vi "build data packet.vi"(0 "Priority (Act immediately)":u8(ring) items=["Act immediately", "Act immediately but disregard errors", "Do not process"], 5 "Timestamp (now)":timestamp, 7 "Metadata":u8[](array[numeric]), 9 "DATA":u8[](array[numeric]), 11 "Footer":u8[](array[numeric])) -> (4 "Byte array":u8[](array[numeric]))   [LabVIEW 2020, in "Template.lvlib" / "Template.lvclass"]
doc: "Builds the data array for the new DVR"
uses:
  Template.lvclass
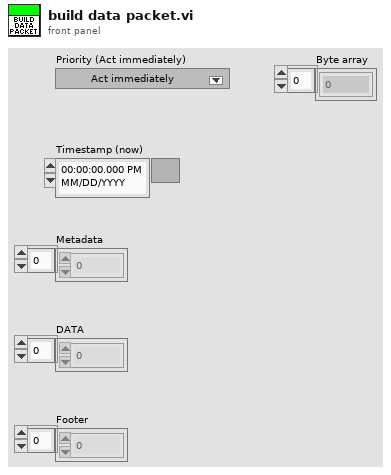
[diagram p1: front panel]
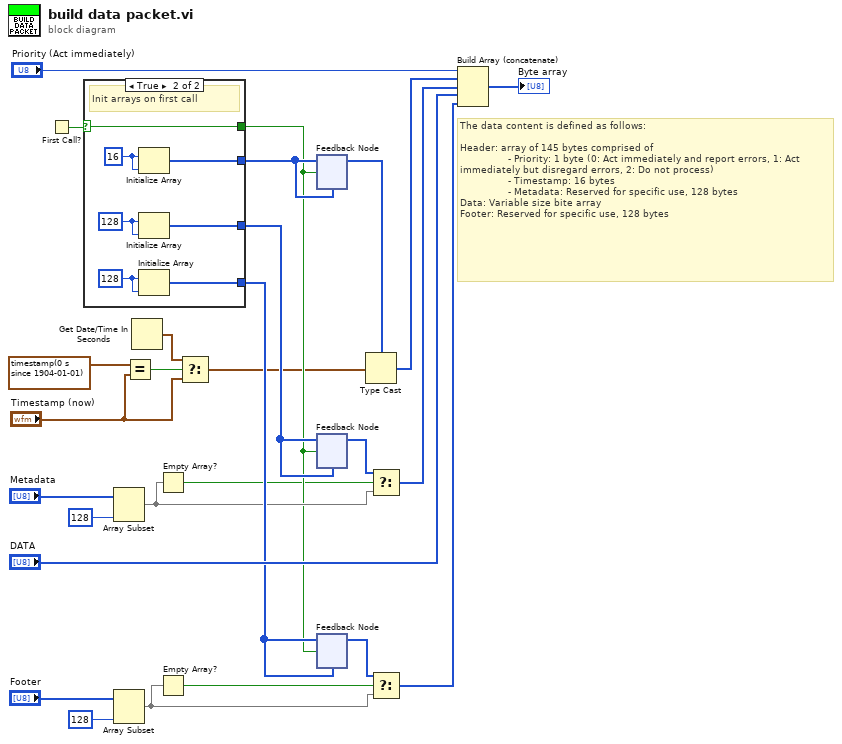
[diagram p0: block diagram]
diagram:
  # "The data content is defined as follows:\n\nHeader: array of 145 bytes comprised of\n                - Priority: 1 byte (0: Act immediately and report errors, 1: Act immediately but disregard errors, 2: Do not process)\n                - Timestamp: 16 bytes\n                - Metadata: Reserved for specific use, 128 bytes\nData: Variable size bite array\nFooter: Reserved for specific use, 128 bytes"
  n1 = First Call?() -> (First Call?: T/F=w23:bool)
  n2 = case shown="True" w23 {
    selector: w23 -> [w28 w33]
    tunnel: [_ w34] -> w24
    tunnel: [w28 w33] -> w7
    tunnel: [_ w30] -> w11
    tunnel: [_ w29] -> w12
    frame False {
      # "Arrays initialized"
    }
    frame True {
      w31 = u8 128 ("Priority (0: act immediately)")
      w32 = u8 128 ("Priority (0: act immediately)")
      w35 = u8 16 ("Priority (0: act immediately)")
      # "Init arrays on first call"
      n3 = Initialize Array(w35, w35) -> (w34:u8[])
      n4 = Initialize Array(w32, w32) -> (w29:u8[])
      n5 = Initialize Array(w31, w31) -> (w30:u8[])
    }
  }
  n6 = Array Subset(array="Metadata", length=128) -> (w9:u8[])  [unwired: 1 in]
  n7 = Array Subset(array="Footer", length=128) -> (w14:u8[])  [unwired: 1 in]
  n8 = Equal?(x=timestamp(0 s since 1904-01-01) ("Timestamp (now)"), y="Timestamp (now)") -> (x = y?=w4:bool)
  n9 = Get Date/Time In Seconds() -> (seconds since 1Jan1904=w3:timestamp)
  n10 = Empty Array?(array=w9) -> (empty?=w6:bool)
  n11 = Empty Array?(array=w14) -> (empty?=w15:bool)
  n12 = Select(t=w3, s=w4, f="Timestamp (now)") -> (s? t:f=w1:timestamp)
  n13 = feedback #1(w24) -> (w25:u8[])
  n14 = feedback-in #1(w24, w7) -> ()
  n15 = feedback #2(w12) -> (w10:u8[])
  n16 = feedback-in #2(w12, w7) -> ()
  n17 = feedback #3(w11) -> (w16:u8[])
  n18 = feedback-in #3(w11, w7) -> ()
  n19 = Type Cast(type=w25, x=w1) -> (*(type *) &x=w26:u8[])
  n20 = Select(t=w10, s=w6, f=w9) -> (s? t:f=w8:u8[])
  n21 = Select(t=w16, s=w15, f=w14) -> (s? t:f=w13:u8[])
  n22 = Build Array (concatenate)("Priority (Act immediately)", w26, w8, "DATA", w13) -> (→"Byte array":u8[])
